vi "替换-TCP连接引用数组元素.vi"(8 "原-连接ID":refnum<k5>, 11 "新-连接ID输入":refnum<k5>) -> (3 "替换成功？":bool)   [LabVIEW 2017]
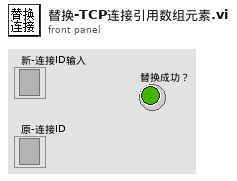
[diagram p1: front panel]
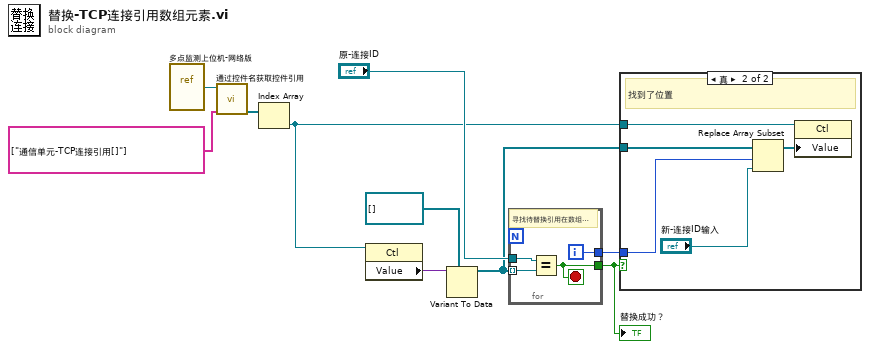
[diagram p0: block diagram]
diagram:
  n1 = vi-ref "多点监测上位机-网络版.vi"() -> (w10:refnum<vi>)
  n2 = call "通过控件名获取控件引用.vi"("控件名数组"=string[] ["通信单元-TCP连接引用[]"], "VI引用"=w10) -> ("控件引用输出"=w8:refnum<vi>[])  [unwired: 7 in, 2 out]
  n3 = Index Array(array=w8) -> (element=w1:refnum<vi>)  [unwired: 1 in]
  n4 = property class="Ctl"(reference=w1) -> ("Value"=w7:variant)  [unwired: 1 in, 2 out]
  n5 = Variant To Data(type=refnum<k5>[] [], Variant=w7) -> (data=w3:refnum<k5>[])  [unwired: 1 in, 1 out]
  n6 = for {
    tunnel: w3 -> [w13] mode=indexing
    tunnel: "原-连接ID" -> [w14]
    tunnel: [w12] -> w4
    tunnel: [w11] -> w2
    i -> [w11]
    stop <- w12 stop-if-true
    # "寻找待替换引用在数组中的位置"
    n7 = Equal?(x=w14, y=w13) -> (x = y?=w12:bool)
  }
  "替换成功？" <- w4
  n8 = case shown="真" w4 {
    tunnel: w3 -> [_ w19]
    tunnel: w2 -> [_ w18]
    tunnel: w1 -> [_ w16]
    frame False {
      # "没找到"
    }
    frame True {
      # "找到了位置"
      n9 = Replace Array Subset(array=w19, new element="新-连接ID输入", index=w18) -> (w15:refnum<k5>[])
      n10 = property class="Ctl"(reference=w16, "Value"=w15) -> ()  [unwired: 1 in, 2 out]
    }
  }
